vi "Add String Setting.vi"(8 "error in":errorcluster, 9 "Initial Value":string, 10 "ID":string, 11 "Controller in":refnum<class "Controller.lvclass">) -> (0 "error out":errorcluster, 3 "Controller out":refnum<class "Controller.lvclass">)   [LabVIEW 2014, in "Controller.lvlib" / "Controller.lvclass"]
uses:
  Controller.lvclass
  Controller.lvclass/Controller.ctl
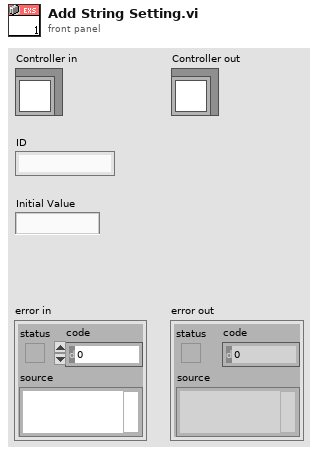
[diagram p1: front panel]
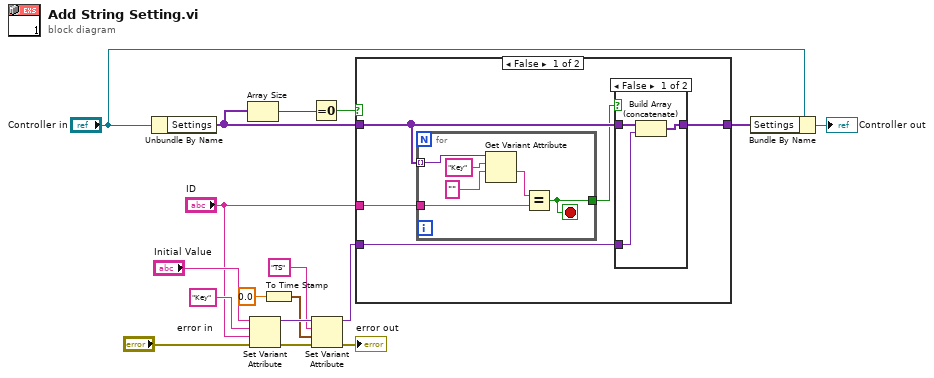
[diagram p0: block diagram]
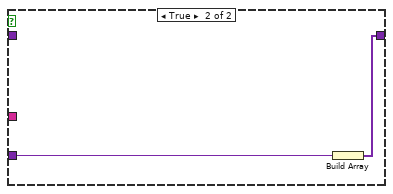
[diagram p3: hidden frame]
diagram:
  n1 = Unbundle By Name("Controller in") -> ("Settings"=w5:variant[])
  n2 = Array Size(array=w5) -> (size(s)=w4:i32)
  n3 = Set Variant Attribute(Variant="Initial Value", name="Key", value="ID", error in="error in") -> (Variant out=w12:variant, error out=w7:errorcluster)  [unwired: 1 out]
  n4 = To Time Stamp(1:0.0) -> (0:w9:timestamp)
  n5 = Equal To 0?(x=w4) -> (x = 0?=w3:bool)
  n6 = Set Variant Attribute(Variant=w12, name="TS", value=w9, error in=w7) -> (Variant out=w11:variant, error out=→"error out":errorcluster)  [unwired: 1 out]
  n7 = case shown="False" w3 {
    tunnel: "ID" -> [w22 _]
    tunnel: w5 -> [w21 _]
    tunnel: [w19 w33] -> w13
    tunnel: w11 -> [w18 w34]
    frame False {
      n8 = for {
        tunnel: w21 -> [w32] mode=indexing
        tunnel: w22 -> [w28]
        tunnel: [w27] -> w20
        stop <- w27 stop-if-true
        n9 = Get Variant Attribute(Variant=w32, name="Key", default value (empty Variant)="") -> (value=w29:string)  [unwired: 1 in, 3 out]
        n10 = Equal?(x=w29, y=w28) -> (x = y?=w27:bool)
      }
      n11 = case shown="False" w20 {
        tunnel: w21 -> [w25 w26]
        tunnel: [w23 w26] -> w19
        tunnel: w18 -> [w24 _]
        frame False {
          n12 = Build Array (concatenate)(w25, w24) -> (w23:variant[])
        }
        frame True {
        }
      }
    }
    frame True {
      n13 = Build Array(w34) -> (w33:variant[])
    }
  }
  n14 = Bundle By Name(cluster="Controller in", "Settings"=w13) -> (→"Controller out":refnum<class "Controller.lvclass">)
